vi "M09 Power Plant.vi"(11 "EV3 in":T1) -> (3 "EV3 out":T1)   [LabVIEW 2016]
uses:
  <vilib>/NXT/Subs/LVHSConnector.ctl
  <vilib>/NXT/LegoClasses/BrickReference/BrickReference.lvclass
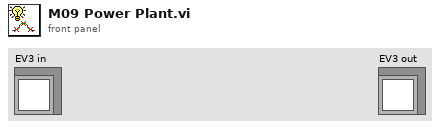
[diagram p1: front panel]
types:
  T1 = typedef "LVHSConnector.ctl" = refnum<class "BrickReference.lvclass">
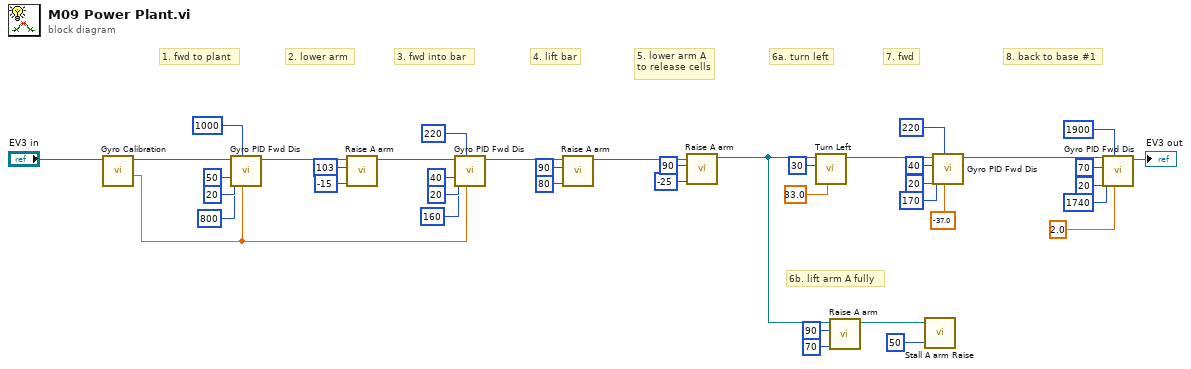
[diagram p0: block diagram]
diagram:
  # "8. back to base #1"
  # "7. fwd"
  # "6b. lift arm A fully"
  # "6a. turn left"
  # "5. lower arm A\nto release cells"
  # "4. lift bar"
  # "3. fwd into bar"
  # "2. lower arm"
  # "1. fwd to plant"
  n1 = call "Gyro Calibration.vi"("NXT/EV3"="EV3 in") -> ("Degrees"=w3:sgl, "NXT/EV3"=w4:T1)  [unwired: 6 in, 1 out]
  n2 = call "Gyro PID Fwd Dis.vi"("Target angle"=w3, "Threshold to stop"=1000, "Threshold to slow"=800, "Min. speed"=20, "Max. speed"=50, "EV3 in"=w4) -> ("EV3 out"=w8:T1)  [unwired: 5 in]
  n3 = call "Raise A arm.vi"("Power"=i8 -15, "Rotation"=103, "EV3 in"=w8) -> ("EV3 out"=w7:T1)  [unwired: 8 in]
  n4 = call "Gyro PID Fwd Dis.vi"("Target angle"=w3, "Threshold to stop"=220, "Threshold to slow"=160, "Min. speed"=20, "Max. speed"=40, "EV3 in"=w7) -> ("EV3 out"=w12:T1)  [unwired: 5 in]
  n5 = call "Raise A arm.vi"("Power"=i8 80, "Rotation"=90, "EV3 in"=w12) -> ("EV3 out"=w6:T1)  [unwired: 8 in]
  n6 = call "Raise A arm.vi"("Power"=i8 -25, "Rotation"=90, "EV3 in"=w6) -> ("EV3 out"=w16:T1)  [unwired: 8 in]
  n7 = call "Turn Left.vi"("Turning angle"=sgl 33.0, "Motor B (right)"=i8 30, "EV3 in"=w16) -> ("EV3 out"=w32:T1)  [unwired: 8 in]
  n8 = call "Raise A arm.vi"("Power"=i8 70, "Rotation"=90, "EV3 in"=w16) -> ("EV3 out"=w18:T1)  [unwired: 8 in]
  n9 = call "Stall A arm Raise.vi"("Power"=i8 50, "NXT/EV3"=w18) -> ()  [unwired: 9 in, 1 out]
  n10 = call "Gyro PID Fwd Dis.vi"("Target angle"=sgl -37.0, "Threshold to stop"=220, "Threshold to slow"=170, "Min. speed"=20 ("Higher speed"), "Max. speed"=40, "EV3 in"=w32) -> ("EV3 out"=w2:T1)  [unwired: 5 in]
  n11 = call "Gyro PID Fwd Dis.vi"("Target angle"=sgl 2.0, "Threshold to stop"=1900, "Threshold to slow"=1740, "Min. speed"=20 ("Higher speed"), "Max. speed"=70, "EV3 in"=w2) -> ("EV3 out"=→"EV3 out":T1)  [unwired: 5 in]
